vi "2DGaussianModel_wRotation.vi"(3 "output control":T1, 4 "data":T2, 5 "X":dbl[](array[numeric]), 6 "a":dbl[](array[numeric])) -> (0 "error out":errorcluster, 1 "f'(X,a)":dbl[][](array[numeric]), 2 "f(X,a)":dbl[](array[numeric]))   [LabVIEW 2016]
doc: "This template is the starting point for creating a model function to be passed to the Nonlinear Curve Fit.vi."
uses:
  <vilib>/gmath/NumericalOptimization/objective function data.ctl
  <vilib>/gmath/NumericalOptimization/LM_output select.ctl
  <vilib>/Analysis/baseanly.llb/A x Vector.vi
  <vilib>/Analysis/Matrix/Numeric/Conversions/Array To Matrix - RA2.vi
  <vilib>/Analysis/Matrix/NI_Matrix.lvlib
  <vilib>/Analysis/NI_AALBase.lvlib
  <vilib>/gmath/NI_Gmath.lvlib
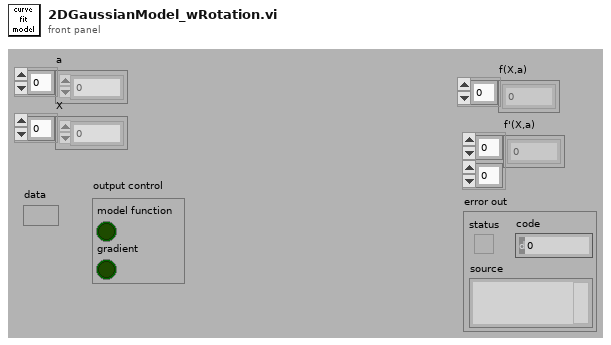
[diagram p1: front panel]
types:
  T1 = typedef "NI_Gmath.lvlib/LM_output select.ctl" = cluster{"model function":bool, "gradient":bool}
  T2 = typedef "NI_Gmath.lvlib/objective function data.ctl" = variant
  T3 = typedef "NI_Matrix.lvlib/RealMatrix.ctl" = dbl[][]
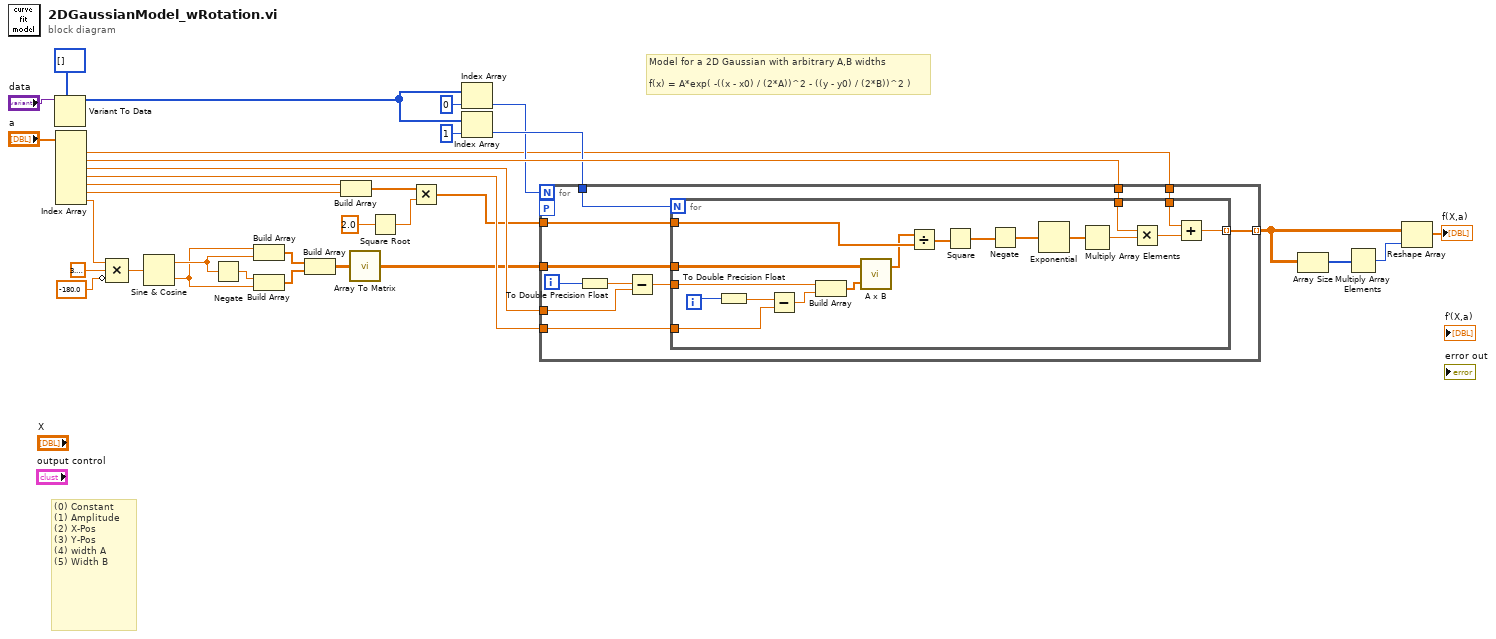
[diagram p0: block diagram]
diagram:
  # "Model for a 2D Gaussian with arbitrary A,B widths\n\nf(x) = A*exp( -((x - x0) / (2*A))^2 - ((y - y0) / (2*B))^2 )"
  # "(0) Constant\n(1) Amplitude\n(2) X-Pos\n(3) Y-Pos\n(4) width A\n(5) Width B"
  n1 = Variant To Data(type=i32[] [], Variant="data") -> (data=w20:i32[])  [unwired: 1 in, 1 out]
  n2 = Index Array(array="a") -> (element #1=w12:dbl, element #2=w19:dbl, element #3=w25:dbl, element #4=w24:dbl, element #5=w30:dbl, element #6=w29:dbl, element #7=w9:dbl)  [unwired: 7 in]
  n3 = Compound Arithmetic op=MULTIPLY(w9, 3.141592653589793, invert -180.0 ("value")) -> (w8:dbl)
  n4 = Sine & Cosine(0:w8) -> (1:w6:dbl, 2:w5:dbl)
  n5 = Negate(x=w6) -> (-x=w7:dbl)
  n6 = Build Array(w5, w6) -> (w4:dbl[])
  n7 = Build Array(w7, w5) -> (w3:dbl[])
  n8 = Build Array(w4, w3) -> (w2:dbl[][])
  n9 = Build Array(w30, w29) -> (w16:dbl[])
  n10 = call-poly <vilib>:"Array To Matrix.vi"("Real 2D Array"=w2) -> ("Real Matrix"=w1:T3)
  n11 = Square Root(x=2.0) -> (sqrt(x)=w14:dbl)
  n12 = Multiply(x=w16, y=w14) -> (x*y=w13:dbl[])
  n13 = Index Array(array=w20, index=0) -> (element=w17:i32)
  n14 = Index Array(array=w20, index=1) -> (element=w18:i32)
  n15 = for {
    N: w17 -> [_]
    tunnel: w13 -> [w44]
    tunnel: [w43] -> w33 mode=indexing
    tunnel: w19 -> [w42]
    tunnel: w18 -> [w41]
    tunnel: w25 -> [w38]
    tunnel: w24 -> [w36]
    workers-P: _ -> [_]
    tunnel: w12 -> [w35]
    tunnel: w1 -> [w34]
    i -> [w40]
    n16 = To Double Precision Float(number=w40) -> (double precision float=w39:dbl)
    n17 = Subtract(x=w39, y=w38) -> (x-y=w37:dbl)
    n18 = for {
      N: w41 -> [_]
      tunnel: w37 -> [w62]
      tunnel: w44 -> [w61]
      tunnel: [w48] -> w43 mode=indexing
      tunnel: w42 -> [w58]
      tunnel: w36 -> [w55]
      tunnel: w35 -> [w49]
      tunnel: w34 -> [w45]
      i -> [w57]
      n19 = To Double Precision Float(number=w57) -> (double precision float=w56:dbl)
      n20 = Subtract(x=w56, y=w55) -> (x-y=w54:dbl)
      n21 = Build Array(w62, w54) -> (w47:dbl[])
      n22 = call-poly <vilib>:"A x B.vi"("Vector"=w47, "A"=w45) -> ("A x Vector"=w46:dbl[])  [unwired: 1 out]
      n23 = Divide(x=w46, y=w61) -> (x/y=w53:dbl[])
      n24 = Square(x=w53) -> (x^2=w52:dbl[])
      n25 = Negate(x=w52) -> (-x=w51:dbl[])
      n26 = Exponential ("Exponential.vi")(1:w51) -> (0:w60:dbl[])
      n27 = Multiply Array Elements(1:w60) -> (0:w59:dbl)
      n28 = Multiply(x=w58, y=w59) -> (x*y=w50:dbl)
      n29 = Add(x=w49, y=w50) -> (x+y=w48:dbl)
    }
  }
  n30 = Array Size(array=w33) -> (size(s)=w31:i32[])
  n31 = Multiply Array Elements(1:w31) -> (0:w32:i32)
  n32 = Reshape Array(w33, w32) -> (→"f(X,a)":dbl[])
